vi "ep_Logarithmic Interpolator.vi"(9 "points":cluster{"x1":dbl, "y1":dbl, "x2":dbl, "y2":dbl}={"x1"=500.0, "y1"=9.0, "x2"=950.0, "y2"=5.0}, 11 "x":dbl=216.66) -> (3 "y":dbl format="%.2f")   [LabVIEW 2011, in "NI_EP_Power Quality.lvlib"]
uses:
  <vilib>/addons/Electrical Power/PQ/NI_EP_Power Quality.lvlib
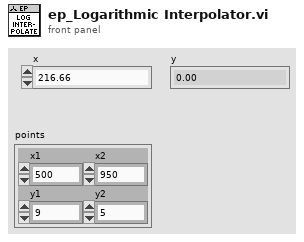
[diagram p1: front panel]
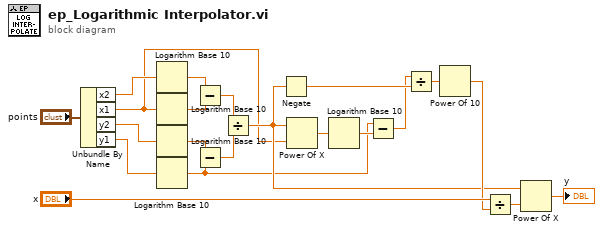
[diagram p0: block diagram]
diagram:
  n1 = Unbundle By Name("points") -> ("x2"=w4:dbl, "x1"=w3:dbl, "y2"=w2:dbl, "y1"=w1:dbl)
  n2 = Logarithm Base 10(1:w4) -> (0:w20:dbl)
  n3 = Logarithm Base 10(1:w3) -> (0:w21:dbl)
  n4 = Logarithm Base 10(1:w2) -> (0:w18:dbl)
  n5 = Logarithm Base 10(1:w1) -> (0:w6:dbl)
  n6 = Subtract(x=w20, y=w21) -> (x-y=w19:dbl)
  n7 = Subtract(x=w18, y=w6) -> (x-y=w17:dbl)
  n8 = Divide(x=w17, y=w19) -> (x/y=w8:dbl)
  n9 = Negate(x=w8) -> (-x=w14:dbl)
  n10 = Power Of X(1:w3, 2:w8) -> (0:w15:dbl)
  n11 = Logarithm Base 10(1:w15) -> (0:w16:dbl)
  n12 = Subtract(x=w6, y=w16) -> (x-y=w13:dbl)
  n13 = Divide(x=w13, y=w14) -> (x/y=w12:dbl)
  n14 = Power Of 10(x=w12) -> (10^x=w9:dbl)
  n15 = Divide(x="x", y=w9) -> (x/y=w11:dbl)
  n16 = Power Of X(1:w11, 2:w8) -> (0:→"y":dbl)
